vi "InspectTell.vi"(6 "Error":errorcluster, 7 "Actor":refnum<class "Actor.lvclass">, 11 "Message":refnum<class "Message.lvclass">) -> (2 "Tell":bool=TRUE, 3 "Message":refnum<class "Message.lvclass">, 4 "Error":errorcluster, 5 "Actor":refnum<class "Actor.lvclass">)   [LabVIEW 2020, in "_Template.lvlib" / "{{Actor}}.lvlib" / "Actor.lvclass"]
uses:
  Actor.lvclass
  jettl/jettl/Message/Message.lvclass
  Actor.lvclass/Actor.ctl
  jettl/jettl/Actor/Actor.lvclass
panel:
  # "This front panel should not be manipulated."
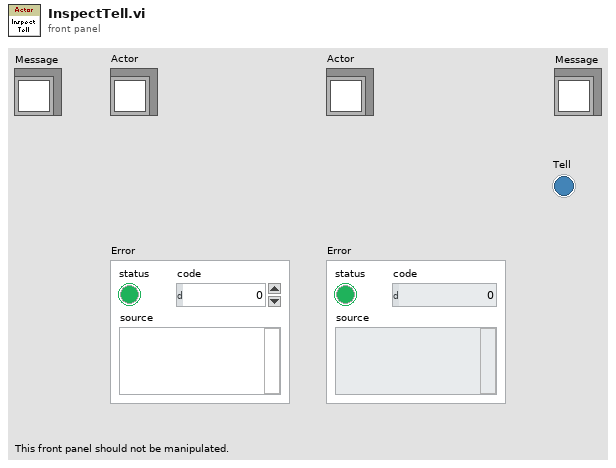
[diagram p1: front panel]
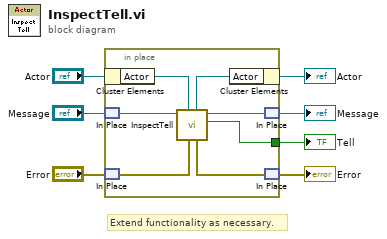
[diagram p0: block diagram]
diagram:
  # "Extend functionality as necessary."
  n1 = in-place {
    in-place-border: [w8] -> w1
    n2 = in-place-cluster #1("Actor") -> ("Actor"=w14:refnum<class "Actor.lvclass">)
    n3 = in-place-match #2("Message") -> (w12:refnum<class "Message.lvclass">)
    n4 = in-place-match #3("Error") -> (w10:errorcluster)
    n5 = call-dynamic "InspectTell.vi"("Error"=w10, "Actor"=w14, "Message"=w12) -> ("Tell"=w8:bool, "Message"=w11:refnum<class "Message.lvclass">, "Error"=w9:errorcluster, "Actor"=w13:refnum<class "Actor.lvclass">)  [unwired: 5 in]
    n6 = in-place-cluster #1("Actor"=w13) -> (→"Actor":refnum<class "Actor.lvclass">)
    n7 = in-place-match #2(w11) -> (→"Message":refnum<class "Message.lvclass">)
    n8 = in-place-match #3(w9) -> (→"Error":errorcluster)
  }
  "Tell" <- w1
